vi "Get Tx Acyclic Execution Time.vi"(8 "error in":errorcluster, 11 "timing section in":T1 format="%.0x") -> (0 "error out":errorcluster, 2 "tx acyclic execution time ref":T1 format="%.0x", 3 "timing section out":T1 format="%.0x")   [LabVIEW 2020, in "Ballard ARINC 429 Scripting.lvlib"]
doc: "Returns all <b>parameters</b> references for the specified <b>label in</b>."
uses:
  Constants.vi
  <vilib>/NI VeriStand/Custom Device Tools/Custom Device Utility Library/NI VeriStand - Search for Item by Name.vi
  Ballard ARINC 429 Scripting.lvlib
  <vilib>/NI VeriStand/Custom Device Tools/Custom Device Utility Library/Custom Device Utility Library.lvlib
  <vilib>/NI VeriStand/Custom Device API/Custom Device Item Ref.ctl
  <vilib>/NI VeriStand/Custom Device API/Custom Device API.lvlib
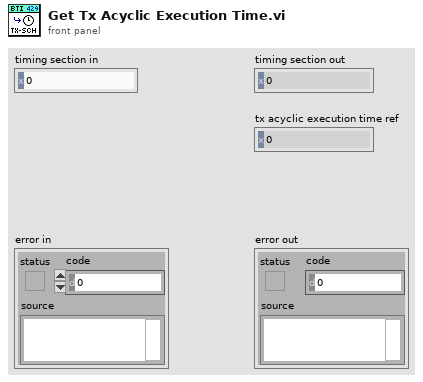
[diagram p1: front panel]
types:
  T1 = typedef "Custom Device API.lvlib/Custom Device Item Ref.ctl" = u64
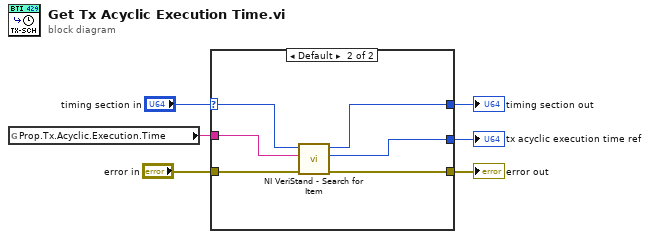
[diagram p0: block diagram]
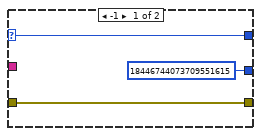
[diagram p2: hidden frame]
diagram:
  n1 = global read "Constants.vi" "Prop.Tx.Acyclic.Execution.Time"() -> (w3:string)
  n2 = case shown="Default" "timing section in" {
    selector: "timing section in" -> [w9 w13]
    tunnel: "error in" -> [w8 w15]
    tunnel: [w9 w14] -> w5
    tunnel: w3 -> [_ w12]
    tunnel: [w8 w11] -> w2
    tunnel: [T1 18446744073709551615 ("Item Ref") w10] -> w1
    frame -1 {
    }
    frame Default {
      n3 = call-poly <vilib>:"NI VeriStand - Search for Item.vi"("error in"=w15, "Item Name"=w12, "Section Ref in"=w13) -> ("error out"=w11:errorcluster, "Item Ref"=w10:T1, "Section Ref out"=w14:T1)  [unwired: 5 in, 1 out]
    }
  }
  "error out" <- w2
  "timing section out" <- w5
  "tx acyclic execution time ref" <- w1
